vi "Configure Output Impedance.vi"(8 "error in (no error)":errorcluster, 9 "impedance (50 Ohms)":dbl[unit]=50.0 format="%.3f", 10 "channel name (\"CHANNEL1\")":string="CHANNEL1", 11 "CS++Fgen in":refnum<class "CS++Fgen.lvclass">) -> (0 "error out":errorcluster, 3 "CS++Fgen out":refnum<class "CS++Fgen.lvclass">)   [LabVIEW 2013, in "CS++Fgen.lvlib" / "CS++Fgen.lvclass"]
doc: "This VI configures the output impedance for the channel you specify."
uses:
  CS++Fgen.lvclass
  Core/Classes/CS++ProcessVariables/ProcessVariable/PV.lvclass
  Core/Classes/CS++ProcessVariables/ProcessVariable/PV.lvclass/PV.ctl
  CS++Fgen.lvclass/CS++Fgen.ctl
  Core/Classes/CS++ProcessVariables/PVConnection/PVConnection.lvclass
  Core/Classes/CS++ProcessVariables/ProcessVariable/Write Data.vi
  Core/Classes/CS++ProcessVariables/ProcessVariable/Write Timestamp.vi
  Core/Classes/CS++ProcessVariables/ProcessVariable/Write Quality.vi
  Core/Classes/CS++ProcessVariables/ProcessVariable/Write status.vi
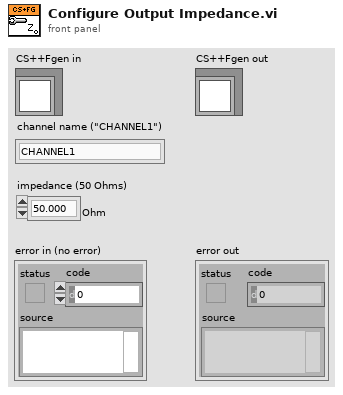
[diagram p1: front panel]
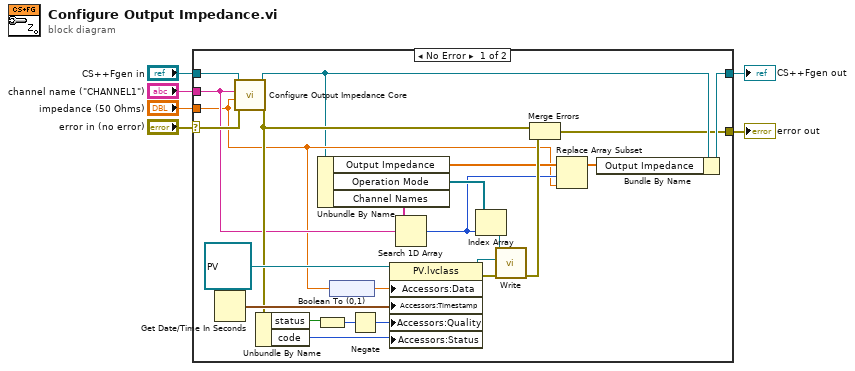
[diagram p0: block diagram]
diagram:
  n1 = case shown="No Error" "error in (no error)" {
    selector: "error in (no error)" -> [w29 w32]
    tunnel: [w8 w32] -> w5
    tunnel: [w9 w31] -> w3
    tunnel: "CS++Fgen in" -> [w30 w31]
    tunnel: "channel name (\"CHANNEL1\")" -> [w12 _]
    tunnel: "impedance (50 Ohms)" -> [w11 _]
    frame No Error {
      n2 = Get Date/Time In Seconds() -> (seconds since 1Jan1904=w28:timestamp)
      n3 = call-dynamic "Configure Output Impedance Core.vi"("error in (no error)"=w29, "impedance (50 Ohms)"=w11, "channel name (\"CHANNEL1\")"=w12, "CS++Fgen in"=w30) -> ("error out"=w13:errorcluster, "CS++Fgen out"=w10:refnum<class "CS++Fgen.lvclass">)  [unwired: 6 in]
      n4 = Unbundle By Name(w13) -> ("status"=w20:bool, "code"=w18:i32)
      n5 = Boolean To (0,1)(Boolean=w20) -> (0, 1=w19:i16)
      n6 = Unbundle By Name(w10) -> ("Output Impedance"=w16:dbl[unit][], "Operation Mode"=w23:refnum<class "PVConnection.lvclass">[], "Channel Names"=w24:string[])
      n7 = node(w11) -> (w7:dbl)
      n8 = Negate(x=w19) -> (-x=w17:i16)
      n9 = property class="PV.lvclass"(reference=refnum<class "PV.lvclass"> refnum ("PV"), "Accessors:Data"=w7, "Accessors:Timestamp"=w28, "Accessors:Quality"=w17, "Accessors:Status"=w18) -> (reference out=w25:refnum<class "PV.lvclass">, error out=w26:errorcluster)  [unwired: 1 in]
      n10 = Search 1D Array(1D array=w24, element=w12) -> (index of element=w14:i32)  [unwired: 1 in]
      n11 = Index Array(array=w23, index=w14) -> (element=w22:refnum<class "PVConnection.lvclass">)
      n12 = call-dynamic "Write.vi"("error in (no error)"=w26, "PV"=w25, "PVConnection in"=w22) -> ("error out"=w21:errorcluster)  [unwired: 7 in, 1 out]
      n13 = Merge Errors(w13, w21) -> (w8:errorcluster)
      n14 = Replace Array Subset(array=w16, new element=w11, index=w14) -> (w15:dbl[unit][])
      n15 = Bundle By Name(cluster=w10, "Output Impedance"=w15) -> (w9:refnum<class "CS++Fgen.lvclass">)
    }
    frame Error {
    }
  }
  "error out" <- w5
  "CS++Fgen out" <- w3
